vi "Main.vi"(8 "error in (no error)":errorcluster, 11 "BMCBase in":refnum<class "BMC.lvclass">) -> (0 "error out":errorcluster, 3 "component":refnum<class "BMC.lvclass">)   [LabVIEW 2012, in "BMC.lvclass"]
doc: "Main VI of the component."
uses:
  BMC.lvclass
  <vilib>/Distrio/Murmex/Murmex/command_enum.ctl
  <vilib>/Distrio/Murmex/InitialiseMessage/InitialiseMessage.lvclass
  <vilib>/Distrio/Murmex/ResetMessage/ResetMessage.lvclass
  <vilib>/Distrio/Murmex/GenericMessage/GenericMessage.lvclass
  <vilib>/Distrio/Murmex/ConfigureMessage/ConfigureMessage.lvclass
  <vilib>/Distrio/Murmex/TerminateMessage/TerminateMessage.lvclass
  <vilib>/Distrio/Murmex/Murmex/update_cluster.ctl
  BMC.lvclass/BMC.ctl
  <vilib>/Distrio/Murmex/Murmex/Set configure at initialise.vi
  <vilib>/Distrio/Murmex/Murmex/Set log reference.vi
  <vilib>/Distrio/Murmex/Murmex/Set VI reference.vi
  <vilib>/Distrio/Murmex/Murmex/Get ID.vi
  <vilib>/Distrio/Murmex/Message/Add or replace parameter.vi
  <vilib>/Distrio/Murmex/Murmex/Murmex.lvclass
  <vilib>/Distrio/Murmex/Message/Message.lvclass
panel:
  in  "Tab Control":T1(tab)
  in  "button: resettomid":bool
  in  "Superactuator":dbl(knob)=50.0 min=0.0 max=300.0 step=1.0 scale=0.0..300.0
  in  "Mirror shape name":string="bob"
  in  "apply superactuator":bool
  in  "apply shape":bool
  in  "button:saveshape":bool
  in  "button: resettoflat":bool
  in  "Load Voltage file":path=path "D:/CLSM_Project/BMC/TestMap1.txt"
  out "DM Voltage Map":dbl[][](graph)
  out "Actuator stats":dbl[][](graph)
  out "log":string
  in  "Component id":string="BMC"
  in  "command":T2
  in  "button:send command":bool
  in  "generic command":string
  in  "button:configure":bool
  in  "button:quit":bool
  out "terminate?":bool
  # "Load voltage map"
  # "Save settings"
  # "Superactuator"
  # "Resets"
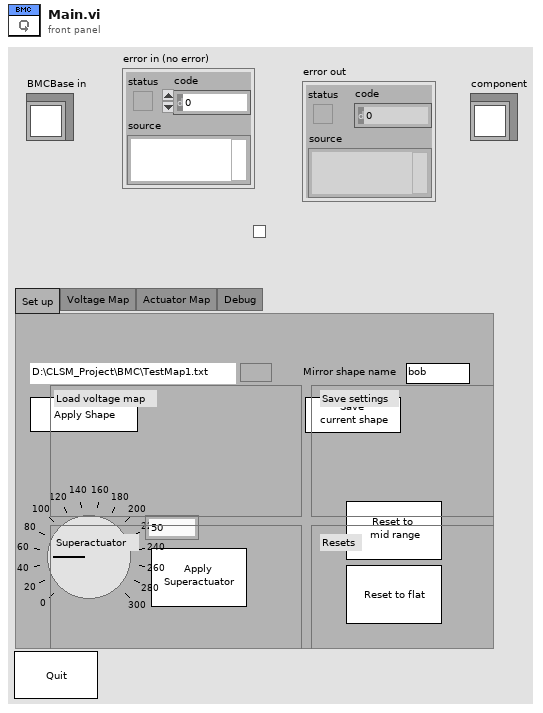
[diagram p1: front panel]
types:
  T1 = enum32{"Set up", "Voltage Map", "Actuator Map", "Debug"}
  T2 = typedef "Murmex.lvlib/Murmex.lvclass/command_enum.ctl" = enum16{"null", "initialise", "reset", "terminate", "acknowledge", "update", "inspect", "inform", "proceed", "start", "stop", "fetch", "configure", "generic"}
  T3 = enum8{"Enabled", "Disabled", "Disabled and Grayed Out"}
  T4 = typedef "Murmex.lvlib/Murmex.lvclass/update_cluster.ctl" = cluster{"target ID":string, "key chains":string[], "values":variant[]}
  T5 = typedef "Murmex.lvclass/command_enum.ctl" = enum16{"null", "initialise", "reset", "terminate", "acknowledge", "update", "inspect", "inform", "proceed", "start", "stop", "fetch", "configure", "generic"}
  T6 = typedef "Murmex.lvclass/Event type enumerations.ctl" = enum16{"before", "after"}
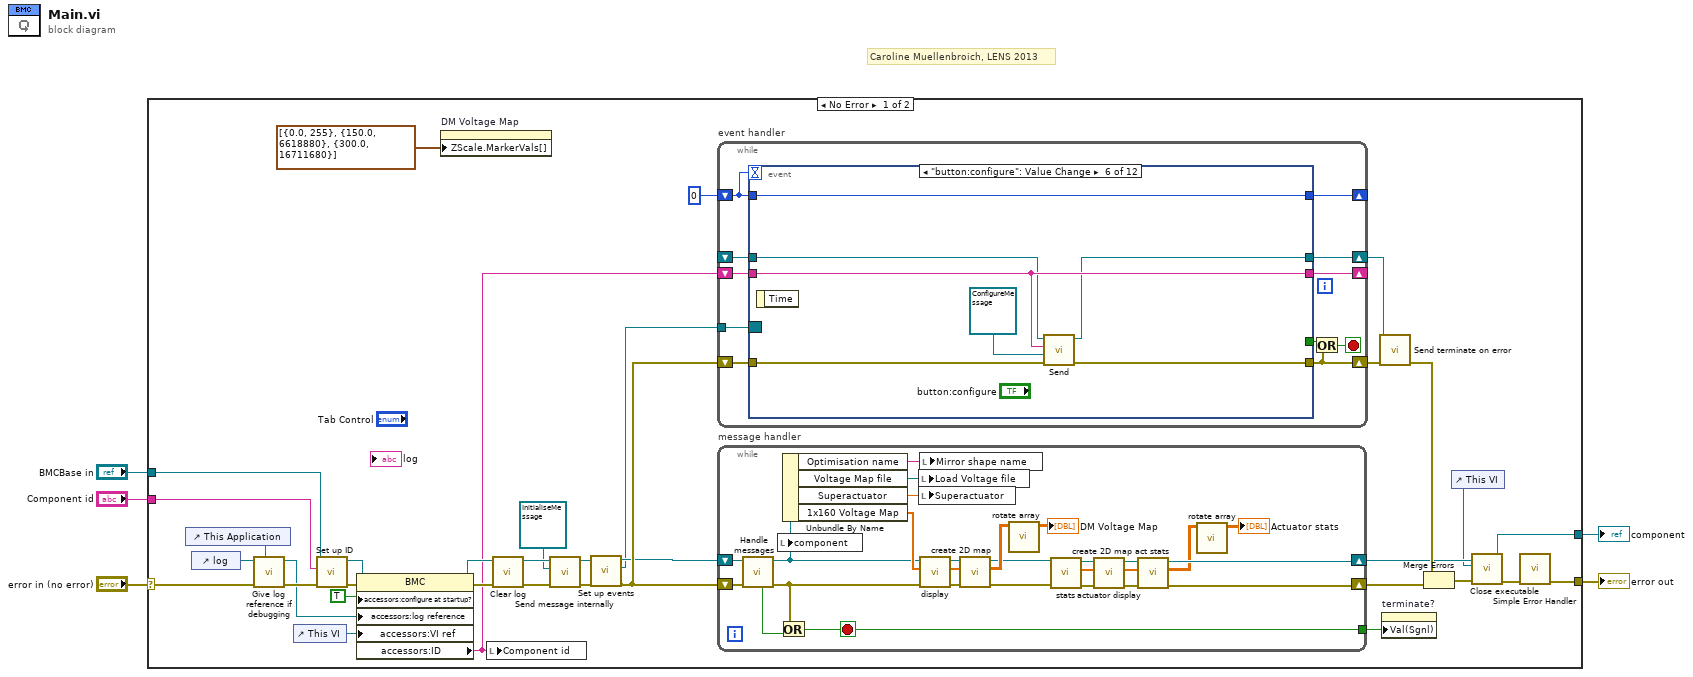
[diagram p0: block diagram]
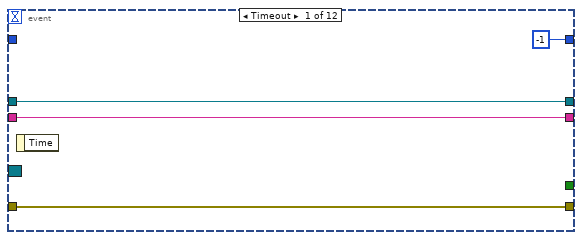
[diagram p2: hidden frame]
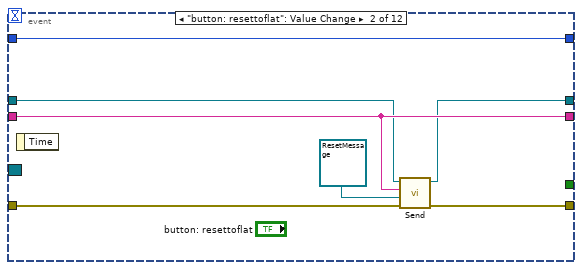
[diagram p3: hidden frame]
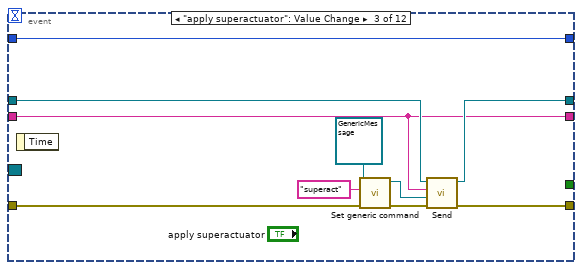
[diagram p4: hidden frame]
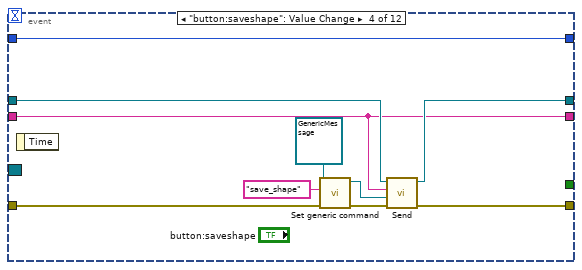
[diagram p5: hidden frame]
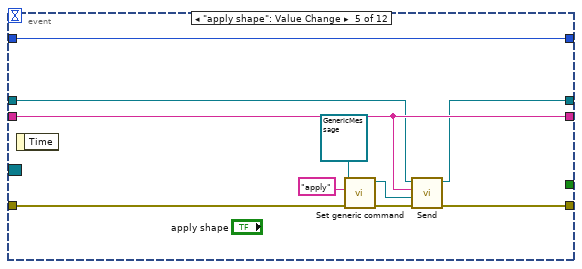
[diagram p6: hidden frame]
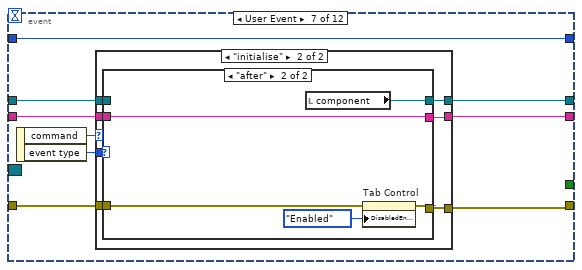
[diagram p7: hidden frame]
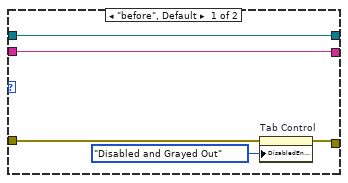
[diagram p9: hidden frame]
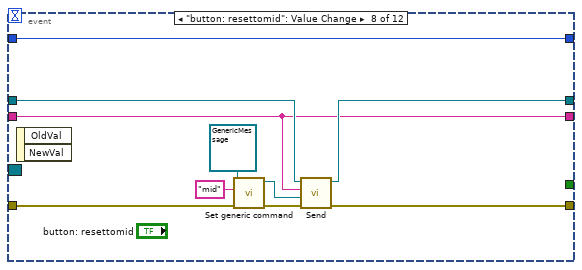
[diagram p10: hidden frame]
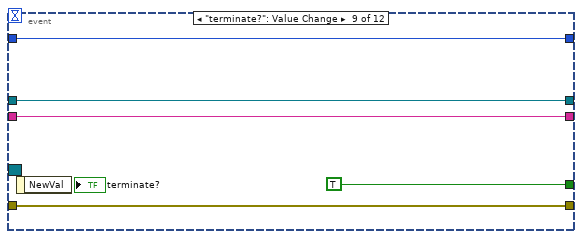
[diagram p11: hidden frame]
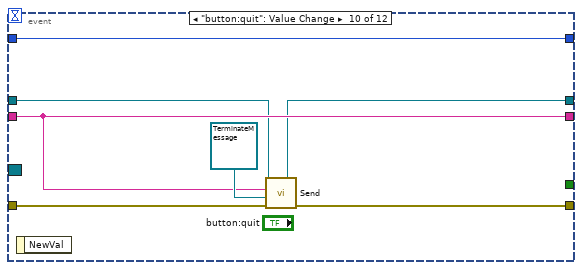
[diagram p12: hidden frame]
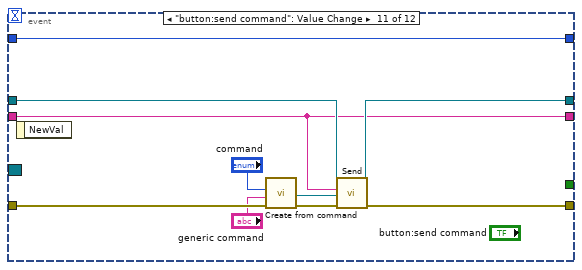
[diagram p13: hidden frame]
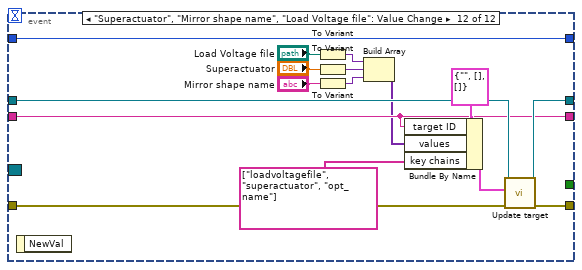
[diagram p14: hidden frame]
diagram:
  # "Caroline Muellenbroich, LENS 2013"
  n1 = case shown="No Error" "error in (no error)" {
    selector: "error in (no error)" -> [w10 w205]
    tunnel: [w15 w204] -> w5
    tunnel: "BMCBase in" -> [w31 w204]
    tunnel: [w16 w205] -> w3
    tunnel: "Component id" -> [w27 _]
    frame No Error {
      n2 = control-ref of="This Application"() -> (w7:refnum<vi>)
      n3 = control-ref of="log"() -> (w8:refnum<vi>)
      n4 = call "Give log reference if debugging.vi"("application ref"=w7, "error in (no error)"=w10, "log reference in"=w8) -> ("error out"=w9:errorcluster, "log reference out"=w6:refnum<vi>)  [unwired: 6 in, 1 out]
      n5 = control-ref of="This VI"() -> (w38:refnum<vi>)
      n6 = call <vilib>:"Set up ID.vi"("error in (no error)"=w9, "component ID"=w27, "MurmexBase in"=w31) -> ("error out"=w32:errorcluster, "MurmexBase out"=w30:refnum<class "BMC.lvclass">)  [unwired: 6 in, 1 out]
      n7 = property class="BMC"(reference=w30, error in=w32, "accessors:configure at startup?"=TRUE ("configure at startup?"), "accessors:log reference"=w6, "accessors:VI ref"=w38) -> (reference out=w40:refnum<class "BMC.lvclass">, error out=w36:errorcluster, "accessors:ID"=w20:string)
      n8 = property on="DM Voltage Map" class="IntGraph (strict)"("ZScale.MarkerVals[]"=cluster{dbl, u32}[] [{0.0, 255}, {150.0, 6618880}, {300.0, 16711680}] ("Z Scale.Marker Values[]")) -> ()  [unwired: 2 in, 2 out]
      n9 = local write "Component id"(w20) -> ()
      n10 = call <vilib>:"Clear log.vi"("error in (no error)"=w36, "MurmexBase in"=w40) -> ("error out"=w35:errorcluster, "MurmexBase out"=w37:refnum<class "BMC.lvclass">)  [unwired: 8 in]
      n11 = call <vilib>:"Send message internally.vi"("error in (no error)"=w35, "Message"=refnum<class "InitialiseMessage.lvclass"> refnum ("InitialiseMessage"), "Murmex in"=w37) -> ("error out"=w26:errorcluster, "Murmex out"=w24:refnum<class "BMC.lvclass">)  [unwired: 7 in]
      n12 = call <vilib>:"Set up events.vi"("error in (no error)"=w26, "MurmexBase in"=w24) -> ("error out"=w25:errorcluster, "Event Registration Refnum"=w22:refnum<event-registration>, "MurmexBase out"=w23:refnum<class "BMC.lvclass">)  [unwired: 7 in]
      n13 = while "event handler" {
        shift-right: [w50] -> w11
        shift-left: w25 -> [w51]
        tunnel: w22 -> [w47]
        shift-right: [w45] -> _
        shift-left: 0 -> [w46]
        shift-right: [w43] -> _
        shift-left: w20 -> [w44]
        shift-right: [w42] -> w12
        shift-left: _ -> [w41]
        stop <- w48 stop-if-true
        n14 = event shown="[5] \"button:configure\": Value Change" {
          selector: w47 -> [_ _ _ _ _ _ _ _ _ _ _ _]
          dyn-events: _ -> [_ _ _ _ _ _ _ _ _ _ _ _]
          timeout: w46 -> [_ _ _ _ _ _ _ _ _ _ _ _]
          tunnel: w51 -> [w55 w57 w67 w78 w88 w99 w106 w131 w143 w148 w160 w174]
          tunnel: [w55 w61 w68 w77 w87 w98 w101 w130 w143 w150 w158 w173] -> w50
          tunnel: [_ _ _ _ _ _ _ _ TRUE _ _ _] -> w49
          tunnel: w46 -> [_ w62 w63 w73 w83 w95 w100 w134 w139 w144 w151 w167]
          tunnel: [-1 w62 w63 w73 w83 w95 w100 w134 w139 w144 w151 w167] -> w45
          tunnel: w44 -> [w53 w60 w64 w74 w86 w96 w105 w129 w141 w147 w152 w169]
          tunnel: [w53 w60 w64 w74 w86 w96 w104 w129 w141 w147 w152 w169] -> w43
          tunnel: [w52 w58 w65 w75 w85 w93 w103 w132 w140 w145 w153 w171] -> w42
          tunnel: w41 -> [w52 w59 w66 w76 w84 w94 w102 w133 w140 w146 w154 w172]
          event Timeout {
            n15 = event-data() -> ()  [unwired: 1 in, 1 out]
          }
          event "button: resettoflat": Value Change {
            n16 = event-data() -> ()  [unwired: 1 in, 1 out]
            n17 = call <vilib>:"Send.vi"("error in (no error)"=w57, "Message"=refnum<class "ResetMessage.lvclass"> refnum ("Message in"), "recipient"=w60, "Murmex in"=w59) -> ("error out"=w61:errorcluster, "Murmex out"=w58:refnum<class "Murmex.lvclass">)  [unwired: 6 in]
          }
          event "apply superactuator": Value Change {
            n18 = event-data() -> ()  [unwired: 1 in, 1 out]
            n19 = call <vilib>:"Set generic command.vi"("error in (no error)"=w67, "generic command"="superact", "GenericMessage in"=refnum<class "GenericMessage.lvclass"> refnum ("GenericMessage")) -> ("error out"=w71:errorcluster, "GenericMessage out"=w70:refnum<class "GenericMessage.lvclass">)  [unwired: 7 in]
            n20 = call <vilib>:"Send.vi"("error in (no error)"=w71, "Message"=w70, "recipient"=w64, "Murmex in"=w66) -> ("error out"=w68:errorcluster, "Murmex out"=w65:refnum<class "Murmex.lvclass">)  [unwired: 6 in]
          }
          event "button:saveshape": Value Change {
            n21 = event-data() -> ()  [unwired: 1 in, 1 out]
            n22 = call <vilib>:"Set generic command.vi"("error in (no error)"=w78, "generic command"="save_shape", "GenericMessage in"=refnum<class "GenericMessage.lvclass"> refnum ("GenericMessage")) -> ("error out"=w81:errorcluster, "GenericMessage out"=w80:refnum<class "GenericMessage.lvclass">)  [unwired: 7 in]
            n23 = call <vilib>:"Send.vi"("error in (no error)"=w81, "Message"=w80, "recipient"=w74, "Murmex in"=w76) -> ("error out"=w77:errorcluster, "Murmex out"=w75:refnum<class "Murmex.lvclass">)  [unwired: 6 in]
          }
          event "apply shape": Value Change {
            n24 = event-data() -> ()  [unwired: 1 in, 1 out]
            n25 = call <vilib>:"Set generic command.vi"("error in (no error)"=w88, "generic command"="apply", "GenericMessage in"=refnum<class "GenericMessage.lvclass"> refnum ("GenericMessage")) -> ("error out"=w91:errorcluster, "GenericMessage out"=w90:refnum<class "GenericMessage.lvclass">)  [unwired: 7 in]
            n26 = call <vilib>:"Send.vi"("error in (no error)"=w91, "Message"=w90, "recipient"=w86, "Murmex in"=w84) -> ("error out"=w87:errorcluster, "Murmex out"=w85:refnum<class "Murmex.lvclass">)  [unwired: 6 in]
          }
          event "button:configure": Value Change {
            n27 = event-data() -> ()  [unwired: 1 in, 1 out]
            n28 = call <vilib>:"Send.vi"("error in (no error)"=w99, "Message"=refnum<class "ConfigureMessage.lvclass"> refnum ("ConfigureMessage"), "recipient"=w96, "Murmex in"=w94) -> ("error out"=w98:errorcluster, "Murmex out"=w93:refnum<class "Murmex.lvclass">)  [unwired: 6 in]
          }
          event User Event {
            n29 = event-data() -> ("command"=w108:T5, "event type"=w107:T6)  [unwired: 1 in]
            n30 = case shown="\"initialise\"" w108 {
              tunnel: w107 -> [_ w118]
              tunnel: w106 -> [w109 w117]
              tunnel: w105 -> [w110 w116]
              tunnel: [w110 w115] -> w104
              tunnel: [w111 w114] -> w103
              tunnel: w102 -> [w111 w113]
              tunnel: [w109 w112] -> w101
              frame "null", Default {
              }
              frame "initialise" {
                n31 = case shown="\"after\"" w118 {
                  tunnel: w117 -> [w120 w128]
                  tunnel: [w119 w126] -> w112
                  tunnel: [w122 w125] -> w115
                  tunnel: w116 -> [w122 w125]
                  tunnel: [w123 w124] -> w114
                  tunnel: w113 -> [w123 _]
                  frame "before", Default {
                    n32 = property on="Tab Control" class="TabCtl (strict)"(error in=w120, "DisabledEnum"=T3."Disabled and Grayed Out" ("Disabled")) -> (error out=w119:errorcluster)  [unwired: 1 in, 1 out]
                  }
                  frame "after" {
                    n33 = local read "component"() -> (w124:refnum<class "BMC.lvclass">)
                    n34 = property on="Tab Control" class="TabCtl (strict)"(error in=w128, "DisabledEnum"=T3."Enabled" ("Disabled")) -> (error out=w126:errorcluster)  [unwired: 1 in, 1 out]
                  }
                }
              }
            }
          }
          event "button: resettomid": Value Change {
            n35 = event-data() -> ()  [unwired: 1 in, 2 out]
            n36 = call <vilib>:"Set generic command.vi"("error in (no error)"=w131, "generic command"="mid", "GenericMessage in"=refnum<class "GenericMessage.lvclass"> refnum ("GenericMessage")) -> ("error out"=w136:errorcluster, "GenericMessage out"=w137:refnum<class "GenericMessage.lvclass">)  [unwired: 7 in]
            n37 = call <vilib>:"Send.vi"("error in (no error)"=w136, "Message"=w137, "recipient"=w129, "Murmex in"=w133) -> ("error out"=w130:errorcluster, "Murmex out"=w132:refnum<class "Murmex.lvclass">)  [unwired: 6 in]
          }
          event "terminate?": Value Change {
            n38 = event-data() -> ()  [unwired: 1 in, 1 out]
          }
          event "button:quit": Value Change {
            n39 = event-data() -> ()  [unwired: 1 in, 1 out]
            n40 = call <vilib>:"Send.vi"("error in (no error)"=w148, "Message"=refnum<class "TerminateMessage.lvclass"> refnum ("TerminateMessage"), "recipient"=w147, "Murmex in"=w146) -> ("error out"=w150:errorcluster, "Murmex out"=w145:refnum<class "Murmex.lvclass">)  [unwired: 6 in]
          }
          event "button:send command": Value Change {
            n41 = event-data() -> ()  [unwired: 1 in, 1 out]
            n42 = call <vilib>:"Create from command.vi"("error in (no error)"=w160, "generic command"="generic command", "command"="command") -> ("error out"=w155:errorcluster, "Message out"=w159:refnum<class "Message.lvclass">)  [unwired: 7 in]
            n43 = call <vilib>:"Send.vi"("error in (no error)"=w155, "Message"=w159, "recipient"=w152, "Murmex in"=w154) -> ("error out"=w158:errorcluster, "Murmex out"=w153:refnum<class "Murmex.lvclass">)  [unwired: 6 in]
          }
          event "Superactuator", "Mirror shape name", "Load Voltage file": Value Change {
            n44 = event-data() -> ()  [unwired: 1 in, 1 out]
            n45 = To Variant(anything="Load Voltage file") -> (Variant=w163:variant)
            n46 = To Variant(anything="Superactuator") -> (Variant=w164:variant)
            n47 = To Variant(anything="Mirror shape name") -> (Variant=w165:variant)
            n48 = Build Array(w163, w164, w165) -> (w168:variant[])
            n49 = Bundle By Name(cluster=T4 {"target ID"="", "key chains"=[], "values"=[]} ("update cluster"), "target ID"=w169, "values"=w168, "key chains"=string[] ["loadvoltagefile", "superactuator", "opt_name"]) -> (w175:T4)
            n50 = call <vilib>:"Update target.vi"("error in (no error)"=w174, "update cluster"=w175, "MurmexBase in"=w172) -> ("error out"=w173:errorcluster, "MurmexBase out"=w171:refnum<class "Murmex.lvclass">)  [unwired: 7 in]
          }
        }
        n51 = Or(x=w49, y=w50) -> (x .or. y?=w48:bool)
      }
      n52 = while "message handler" {
        shift-right: [w188] -> w29
        shift-left: w25 -> [w203]
        shift-right: [w184] -> w14
        shift-left: w23 -> [w200]
        tunnel: [w201] -> w33
        stop <- w201 stop-if-true
        n53 = call <vilib>:"Handle messages.vi"("error in (no error)"=w203, "Murmex in"=w200) -> ("error out"=w197:errorcluster, "Murmex out"=w180:refnum<class "BMC.lvclass">, "terminated?"=w202:bool)  [unwired: 7 in]
        n54 = local write "component"(w180) -> ()
        n55 = Or(x=w197, y=w202) -> (x .or. y?=w201:bool)
        n56 = Unbundle By Name(w180) -> ("Optimisation name"=w177:string, "Voltage Map file"=w178:path, "Superactuator"=w179:dbl, "1x160 Voltage Map"=w196:dbl[])
        n57 = local write "Load Voltage file"(w178) -> ()
        n58 = local write "Superactuator"(w179) -> ()
        n59 = local write "Mirror shape name"(w177) -> ()
        n60 = call "display.vi"("error in (no error)"=w197, "1x160 Voltage Map"=w196, "BMC in"=w180) -> ("error out"=w192:errorcluster, "1x160 Voltage Map 2"=w191:dbl[], "BMC out"=w193:refnum<class "BMC.lvclass">)  [unwired: 6 in]
        n61 = call-dynamic "create 2D map.vi"("error in (no error)"=w192, "Voltage array"=w191, "BMC in"=w193) -> ("error out"=w189:errorcluster, "2D Voltage Map"=w198:dbl[][], "BMC out"=w187:refnum<class "BMC.lvclass">)  [unwired: 6 in]
        n62 = call "rotate array.vi"("Array 2"=w198) -> ("Array"=→"DM Voltage Map":dbl[][])  [unwired: 10 in]
        n63 = call-dynamic "stats.vi"("error in (no error)"=w189, "BMC in"=w187) -> ("error out"=w195:errorcluster, "actuator array"=w194:dbl[], "BMC out"=w186:refnum<class "BMC.lvclass">)  [unwired: 7 in]
        n64 = call "actuator display.vi"("error in (no error)"=w195, "actuator array in"=w194, "BMC in"=w186) -> ("error out"=w190:errorcluster, "actuator array out"=w181:dbl[], "BMC out"=w185:refnum<class "BMC.lvclass">)  [unwired: 6 in]
        n65 = call-dynamic "create 2D map act stats.vi"("error in (no error)"=w190, "Actuator array in"=w181, "BMC in"=w185) -> ("error out"=w188:errorcluster, "actuator stats out"=w182:dbl[][], "BMC out"=w184:refnum<class "BMC.lvclass">)  [unwired: 6 in]
        n66 = call "rotate array.vi"("Array 2"=w182) -> ("Array"=→"Actuator stats":dbl[][])  [unwired: 10 in]
      }
      n67 = call <vilib>:"Send terminate on error.vi"("error in (no error)"=w11, "Murmex in"=w12) -> ("error out"=w19:errorcluster)  [unwired: 8 in, 1 out]
      n68 = property on="terminate?" class="Bool (strict)"("Val(Sgnl)"=w33) -> ()  [unwired: 2 in, 2 out]
      n69 = Merge Errors(w19, w29) -> (w17:errorcluster)
      n70 = control-ref of="This VI"() -> (w13:refnum<vi>)
      n71 = call <vilib>:"Close executable.vi"("error in (no error)"=w17, "main VI ref (optional)"=w13, "MurmexBase in"=w14) -> ("error out"=w18:errorcluster, "MurmexBase out"=w15:refnum<class "BMC.lvclass">)  [unwired: 7 in]
      n72 = call <vilib>:"Simple Error Handler.vi"("error in (no error)"=w18) -> ("error out"=w16:errorcluster)  [unwired: 4 in, 4 out]
    }
    frame Error {
    }
  }
  "error out" <- w3
  "component" <- w5
